vi "p11 imagen a gris.vi"() -> ()   [LabVIEW 2013]
panel:
  out "new picture":picture
  in  "path":path
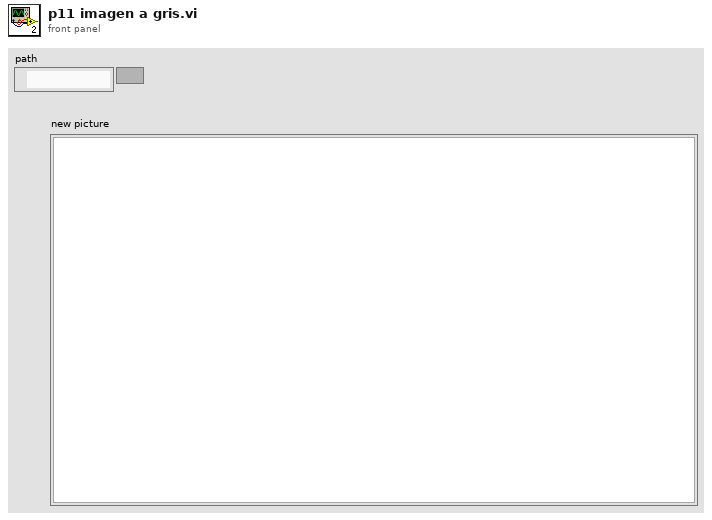
[diagram p1: front panel]
types:
  T1 = typedef "imagedata.ctl" = cluster{"image type":i32, "image depth":i32, "image":u8[], "mask":u8[], "colors":u32[], "Rectangle":cluster{"left":i16, "top":i16, "right":i16, "bottom":i16}}
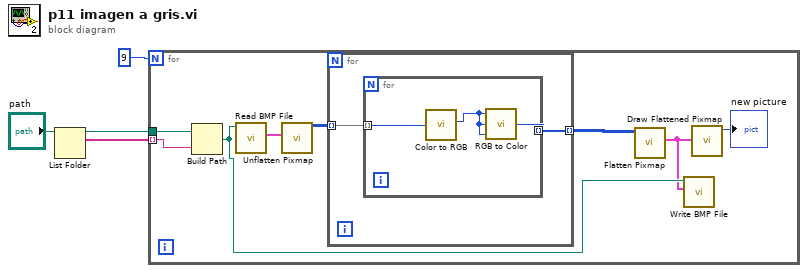
[diagram p0: block diagram]
diagram:
  n1 = List Folder(path="path") -> (path out=w3:path, filenames=w2:string[])  [unwired: 3 in, 2 out]
  n2 = for {
    N: 9 -> [_]
    tunnel: w3 -> [w12]
    tunnel: w2 -> [w11] mode=indexing
    n3 = Build Path(base path=w12, name or relative path=w11) -> (appended path=w6:path)
    n4 = call <vilib>:"Read BMP File.vi"("path to BMP file"=w6) -> ("image data"=w10:T1)  [unwired: 8 in, 2 out]
    n5 = call <vilib>:"Unflatten Pixmap.vi"("image data"=w10) -> ("24-bit pixmap"=w9:u32[][])  [unwired: 4 in, 6 out]
    n6 = for {
      tunnel: w9 -> [w14] mode=indexing
      tunnel: [w13] -> w8 mode=indexing
      n7 = for {
        tunnel: w14 -> [w17] mode=indexing
        tunnel: [w16] -> w13 mode=indexing
        n8 = call <vilib>:"Color to RGB.vi"("Color"=w17) -> ("R"=w15:u8)  [unwired: 3 out]
        n9 = call <vilib>:"RGB to Color.vi"("B"=w15, "G"=w15, "R"=w15) -> ("Color"=w16:u32)
      }
    }
    n10 = call <vilib>:"Flatten Pixmap.vi"("24-bit pixmap"=w8) -> ("image data"=w5:T1)  [unwired: 10 in]
    n11 = call <vilib>:"Write BMP File.vi"("image data"=w5, "path to BMP file"=w6) -> ()  [unwired: 8 in, 2 out]
    n12 = call <vilib>:"Draw Flattened Pixmap.vi"("image data"=w5) -> ("new picture"=→"new picture":picture)  [unwired: 8 in]
  }
